vi "Pack Mission Mission Settings Message.vi"(11 "Mission Controller Settings":T1) -> (3 "Set Mission Controller Settings Message out":refnum<class "Set Mission Controller Settings Message.lvclass">)   [LabVIEW 2015, in "RDS Mission Controller Actor.lvlib"]
uses:
  RDS Mission Controller Actor.lvlib
  Mission Controller Settings.ctl
  Libraries/RDS Child Messages/Mission Messages/Set Mission Controller Settings Message.lvclass
  Libraries/RDS Framework/RDS Message ID.ctl
  Libraries/RDS Framework/RDS Message Class/RDS Message.lvclass/RDS Message.ctl
  Libraries/RDS Child Messages/Mission Messages/Set Mission Controller Settings Message.lvclass/Set Mission Controller Settings Message.ctl
  Libraries/RDS Framework/RDS Message Class/RDS Message.lvclass
  Libraries/RDS Child Messages/RDS Child Messages.lvlib
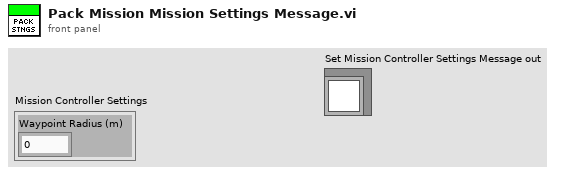
[diagram p1: front panel]
types:
  T1 = typedef "RDS Mission Controller Actor.lvlib/Mission Controller Settings.ctl" = cluster{"Waypoint Radius (m)":dbl}
  T2 = typedef "RDS Child Messages.lvlib/RDS Message ID.ctl" = enum16{"RDS Hello World", "String Message", "AIP_Status", "AIP_Command", "GPS_Data", "MCB_Command", "MCB_Status", "Compass_Data", "Depth_Data", "Battery_Data", "Contoller_State", "Set_Mag_Dev", "BTB_Shutdown", "State_Sample_Request", "State_Sample", "PID_Gains_Set", "Helm_Limiter_Set", "Helm_Heading_Command", "Helm_Steering_Command", "Helm_Status", "Controller_Message", "AIP_Set_Min_Depth", "Mission_Controller_State", "Mission_Upload", "Mission_Set_Op_and_Run", "Mission_Settings_Set"}
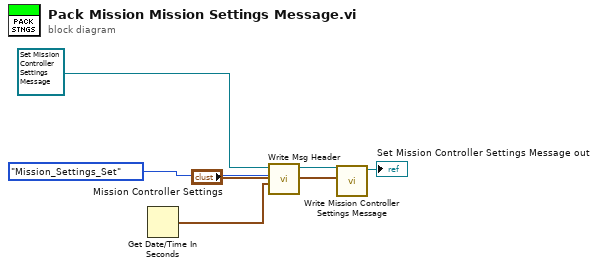
[diagram p0: block diagram]
diagram:
  n1 = Get Date/Time In Seconds() -> (seconds since 1Jan1904=w6:timestamp)
  n2 = call "Write Msg Header.vi"("Time Stamp"=w6, "Msg ID"=RDS_Message_ID."Mission_Settings_Set", "RDS Message in"=refnum<class "Set Mission Controller Settings Message.lvclass"> refnum ("RDS Child Messages.lvlib:Set Mission Controller Settings Message.lvclass")) -> ("RDS Message out"=w3:refnum<class "Set Mission Controller Settings Message.lvclass">)  [unwired: 7 in, 1 out]
  n3 = call "Write Mission Controller Settings Message.vi"("Mission Controller Settings"="Mission Controller Settings", "Set Mission Controller Settings Message in"=w3) -> ("Set Mission Controller Settings Message out"=→"Set Mission Controller Settings Message out":refnum<class "Set Mission Controller Settings Message.lvclass">)  [unwired: 8 in, 1 out]
